vi "transform.vi"(6 "SpaceVector.lvclass":refnum<class "SpaceVector.lvclass">, 7 "zoom":dbl, 8 "error in (no error)":errorcluster, 9 "x angle (psi)":dbl[unit], 10 "z angle (phi)":dbl[unit], 11 "TrajectoryMG100122AODFrameScan in":refnum<class "TrajectoryMH100122AODRAPS.lvclass">) -> (0 "error out":errorcluster, 3 "TrajectoryMG100122AODFrameScan out":refnum<class "TrajectoryMH100122AODRAPS.lvclass">)   [LabVIEW 2010, in "TrajectoryMH100122AODRAPS.lvclass"]
uses:
  TrajectoryMH100122AODRAPS.lvclass
  common/classes/SpaceVector/SpaceVector/SpaceVector.lvclass
  TrajectoryMG100122GenericFPGA/TrajectoryMG100122GenericFPGA/TrajectoryMG100122GenericFPGA.lvclass
  FPGAWrapper/FPGAWrapperMH120124AOD/FPGAWrapperMH120124RAPS_PXI7813R/FPGAWrapperMH120124RAPS_PXI7813R.lvclass
  FPGAWrapper/GenericFPGAWrapper/GenericFPGAWrapper/GenericFPGAWrapper.lvclass
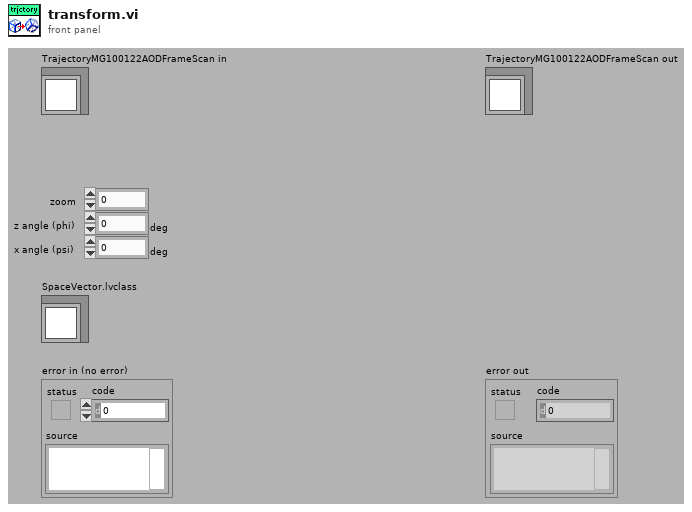
[diagram p1: front panel]
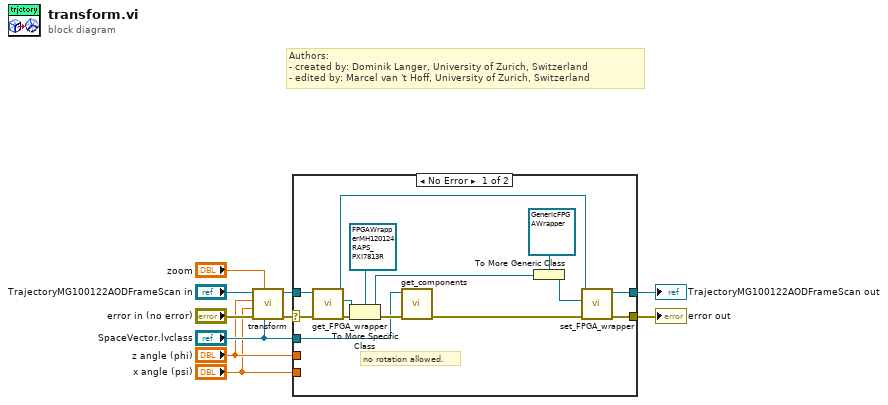
[diagram p0: block diagram]
diagram:
  # "Authors: \n- created by: Dominik Langer, University of Zurich, Switzerland\n- edited by: Marcel van 't Hoff, University of Zurich, Switzerland"
  n1 = call-parent "transform.vi"("SpaceVector.lvclass"="SpaceVector.lvclass", "zoom"="zoom", "error in (no error)"="error in (no error)", "x angle (psi)"="x angle (psi)", "z angle (phi)"="z angle (phi)", "TrajectoryMG100122GenericFPGA in"="TrajectoryMG100122AODFrameScan in") -> ("error out"=w8:errorcluster, "TrajectoryMG100122GenericFPGA out"=w7:refnum<class "TrajectoryMH100122AODRAPS.lvclass">)  [unwired: 4 in]
  n2 = case shown="No Error" w8 {
    selector: w8 -> [w23 w25]
    tunnel: w7 -> [w24 w26]
    tunnel: "SpaceVector.lvclass" -> [w19 _]
    tunnel: "z angle (phi)" -> [_ _]
    tunnel: "x angle (psi)" -> [_ _]
    tunnel: [w18 w25] -> w2
    tunnel: [w16 w26] -> w1
    frame No Error {
      # "no rotation allowed."
      n3 = call-dynamic "get_FPGA_wrapper.vi"("error in (no error)"=w23, "TrajectoryMG100122GenericFPGA in"=w24) -> ("error out"=w21:errorcluster, "GenericFPGAWrapper.lvclass"=w22:refnum<class "GenericFPGAWrapper.lvclass">, "TrajectoryMG100122GenericFPGA out"=w17:refnum<class "TrajectoryMH100122AODRAPS.lvclass">)  [unwired: 7 in]
      n4 = To More Specific Class(target class=refnum<class "FPGAWrapperMH120124RAPS_PXI7813R.lvclass"> refnum ("FPGAWrapperMH120124RAPS_PXI7813R.lvclass"), reference=w22, error in=w21) -> (specific class reference=w12:refnum<class "FPGAWrapperMH120124RAPS_PXI7813R.lvclass">, error out=w20:errorcluster)
      n5 = call "get_components.vi"("error in (no error)"=w20, "SpaceVector in"=w19) -> ("error out"=w11:errorcluster)  [unwired: 4 in, 5 out]
      n6 = To More Generic Class(target class=refnum<class "GenericFPGAWrapper.lvclass"> refnum ("GenericFPGAWrapper.lvclass"), reference=w12) -> (generic class reference=w15:refnum<class "GenericFPGAWrapper.lvclass">)
      n7 = call-dynamic "set_FPGA_wrapper.vi"("error in (no error)"=w11, "GenericFPGAWrapper.lvclass"=w15, "TrajectoryMG100122GenericFPGA in"=w17) -> ("error out"=w18:errorcluster, "TrajectoryMG100122GenericFPGA out"=w16:refnum<class "TrajectoryMH100122AODRAPS.lvclass">)  [unwired: 7 in]
    }
    frame Error {
    }
  }
  "error out" <- w2
  "TrajectoryMG100122AODFrameScan out" <- w1
